vi "test harness_FXP_Linear_control_law.vi"(8 "error in (no error)":errorcluster, 11 "TestCase in":refnum<class "FXP_observer_TestCase.lvclass">) -> (0 "error out":errorcluster, 3 "TestCase out":refnum<class "FXP_observer_TestCase.lvclass">)   [LabVIEW 2017, in "FXP_observer_TestCase.lvclass"]
uses:
  FXP_observer_TestCase.lvclass
  <vilib>/rvi/DesktopExecutionNode/DesktopExecutionNode.xnode
  <vilib>/rvi/DesktopExecutionNode/Execution/niFpgaDEN_Execute.vi
  fpga_VIs/fpga_subVIs_ssxy/fixed-point-ss/typeDefs/FXPControlParams_distEst.ctl
panel:
  in  "ControlParams_distEst 2":T1={"umax"=3.0, "Ns_obs/cntrl"=22, "ref_f_VEC"=[0.0, 0.0], "du_max"=5.0, "Nbar"=0.0}
  out "xerr(expected)":fxp<+/-,64,11>[](array[numeric])
  out "x*y":fxp<+/-,64,10>[](array[numeric])
  out "xerr":fxp<+/-,32,8>[](array[numeric])
  in  "yd_est":fxp<+/-,32,5>
  out "error (xerr)":errorcluster
  out "delta uk (expected)":dbl
  out "del u(k)":fxp<+/-,64,15>
  out "error (delta uk)":errorcluster
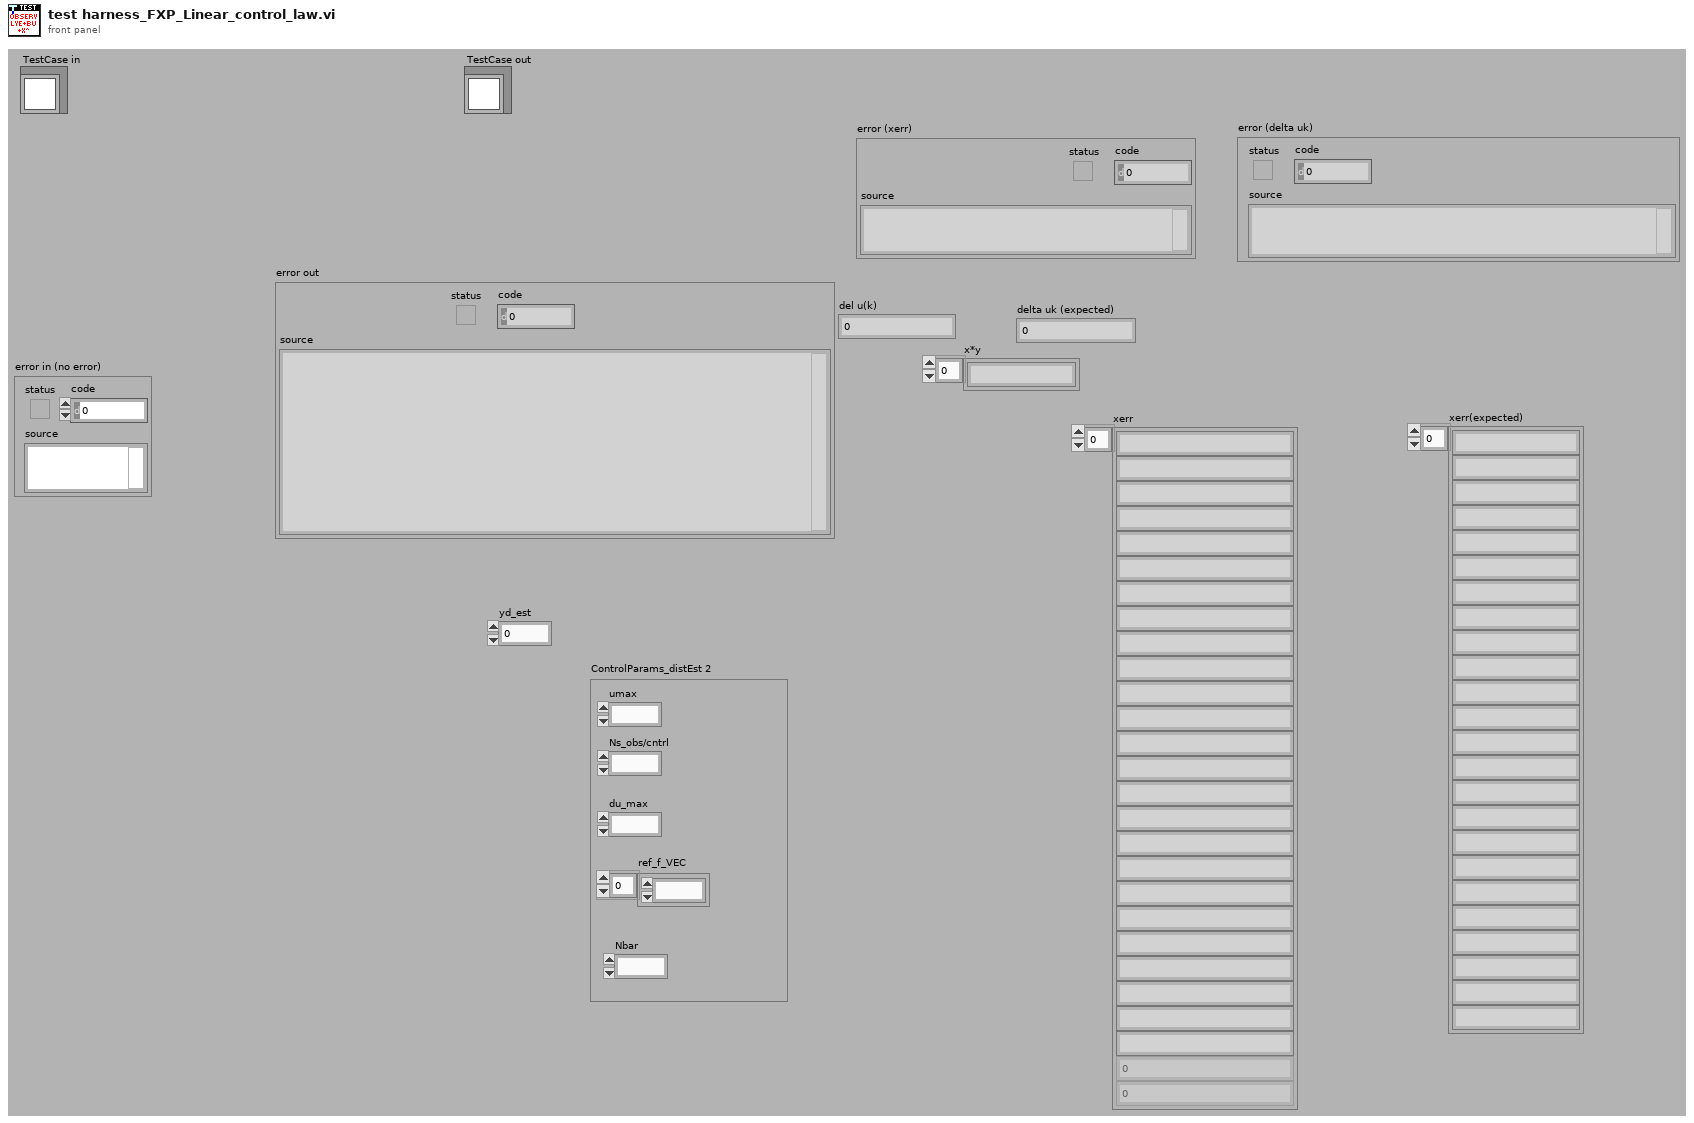
[diagram p1: front panel]
types:
  T1 = typedef "FXPControlParams_distEst.ctl" = cluster{"umax":fxp<+/-,18,5>, "Ns_obs/cntrl":u8, "ref_f_VEC":fxp<+/-,32,5>[], "du_max":fxp<+/-,18,5>, "Nbar":fxp<+/-,18,5>}
  T2 = typedef "UT_matrix_data.ctl" = cluster{"Bz":T3[], "Ldist":T4[], "Kz":T5[], "Nx":T6[], "Ax_col":T7[], "X_vec":T8[], "Cz":T9[]}
  T3 = typedef "Bz_vec_scalar.ctl" = fxp<+/-,32,3>
  T4 = typedef "Lz_vec_scalar.ctl" = fxp<+/-,32,3>
  T5 = typedef "Kz_vec_scalar.ctl" = fxp<+/-,32,10>
  T6 = typedef "Nx_vec_scalar.ctl" = fxp<+/-,32,2>
  T7 = typedef "Az_vec_scalar.ctl" = fxp<+/-,32,7>
  T8 = typedef "x_vec_scalar.ctl" = fxp<+/-,32,6>
  T9 = typedef "Cz_vec_scalar.ctl" = fxp<+/-,32,4>
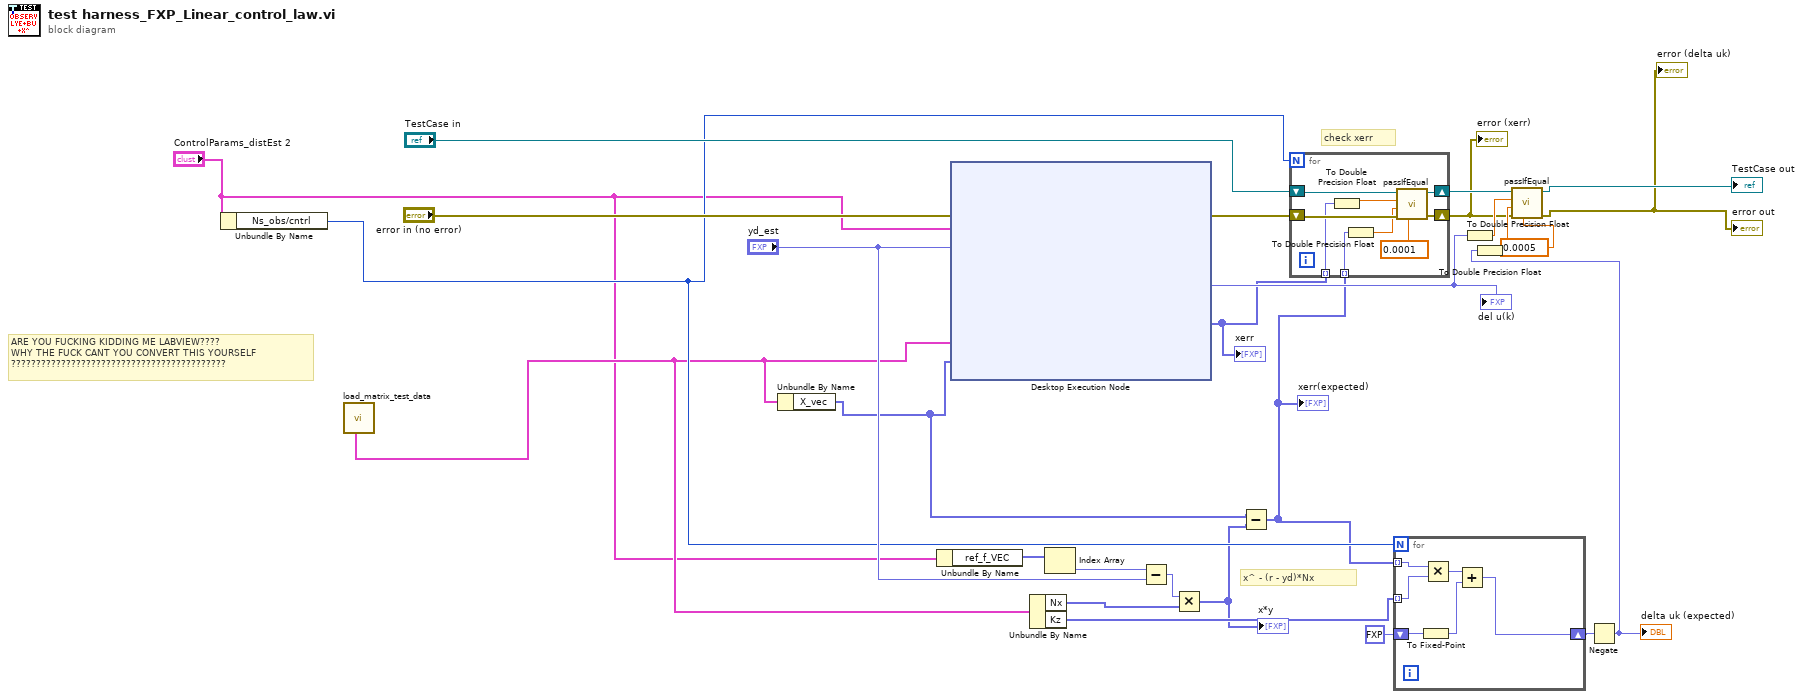
[diagram p0: block diagram]
diagram:
  # "x^ - (r - yd)*Nx"
  # "check xerr"
  # "ARE YOU FUCKING KIDDING ME LABVIEW????\nWHY THE FUCK CANT YOU CONVERT THIS YOURSELF\n???????????????????????????????????????????"
  n1 = Unbundle By Name("ControlParams_distEst 2") -> ("Ns_obs/cntrl"=w8:u8)
  n2 = call "load_matrix_test_data.vi"() -> ("output cluster"=w2:T2)  [unwired: 4 in, 7 out]
  n3 = Unbundle By Name(w2) -> ("X_vec"=w4:T8[])
  n4 = Unbundle By Name("ControlParams_distEst 2") -> ("ref_f_VEC"=w24:fxp<+/-,32,5>[])
  n5 = xnode "Desktop Execution Node"("Error In"="error in (no error)", "ControlParams_distEst"="ControlParams_distEst 2", "yd_est"="yd_est", "Matrix Data"=w2, "xk_12"=w4) -> ("Error Out"=w18:errorcluster, "del u(k)"=w12:fxp<+/-,64,15>, "xerr"=w3:fxp<+/-,32,6>[])  [unwired: 2 out]
  "del u(k)" <- w12
  "xerr" <- w3
  n6 = Unbundle By Name(w2) -> ("Nx"=w25:T6[], "Kz"=w22:T5[])
  n7 = Index Array(array=w24) -> (element=w23:fxp<+/-,32,5>)  [unwired: 1 in]
  n8 = Subtract(x=w23, y="yd_est") -> (x-y=w26:fxp<+/-,32,5>)
  n9 = Multiply(x=w26, y=w25) -> (x*y=w5:fxp<+/-,64,10>[])
  "x*y" <- w5
  n10 = Subtract(x=w4, y=w5) -> (x-y=w6:T8[])
  "xerr(expected)" <- w6
  n11 = for {
    N: w8 -> [_]
    shift-right: [w36] -> w16
    shift-left: "TestCase in" -> [w33]
    shift-right: [w35] -> w9
    shift-left: w18 -> [w34]
    tunnel: w6 -> [w30] mode=indexing
    tunnel: w3 -> [w29] mode=indexing
    n12 = To Double Precision Float(number=w29) -> (double precision float=w31:dbl)
    n13 = To Double Precision Float(number=w30) -> (double precision float=w32:dbl)
    n14 = call-dynamic "passIfEqual.vi"("delta (optional)"=0.0001 ("del u_x"), "error in (no error)"=w34, "y"=w32, "x"=w31, "TestCase in"=w33) -> ("error out"=w35:errorcluster, "TestCase out"=w36:refnum<class "FXP_observer_TestCase.lvclass">)  [unwired: 5 in]
  }
  "error (xerr)" <- w9
  n15 = for {
    N: w8 -> [_]
    tunnel: w6 -> [w42] mode=indexing
    tunnel: w22 -> [w41] mode=indexing
    shift-right: [w39] -> w20
    shift-left: fxp<+,32,5> 0.0 -> [w38]
    n16 = To Fixed-Point(number=w38) -> (fixed-point=w37:fxp<+/-,64,15>)  [unwired: 1 in]
    n17 = Multiply(x=w42, y=w41) -> (x*y=w40:fxp<+/-,64,16>)
    n18 = Add(x=w40, y=w37) -> (x+y=w39:fxp<+/-,64,16>)
  }
  n19 = To Double Precision Float(number=w12) -> (double precision float=w15:dbl)
  n20 = Negate(x=w20) -> (-x=w13:fxp<+/-,64,17>)
  "delta uk (expected)" <- w13
  n21 = To Double Precision Float(number=w13) -> (double precision float=w14:dbl)
  n22 = call-dynamic "passIfEqual.vi"("delta (optional)"=0.0005 ("del u_x"), "error in (no error)"=w9, "y"=w14, "x"=w15, "TestCase in"=w16) -> ("error out"=→"error out" →"error (delta uk)":errorcluster, "TestCase out"=→"TestCase out":refnum<class "FXP_observer_TestCase.lvclass">)  [unwired: 5 in]
